vi "NumArray_to_SpdshtStr.vi"(10 "element 2":dbl[](array[numeric]), 11 "element":dbl[](array[numeric])) -> (1 "concatenated string":string, 2 "XY Graph":T1(graph))   [LabVIEW 2015]
panel:
  in  "delimiter (Tab) 2":string
  in  "Column headers":string[](array[string])
  out "spreadsheet string":string
  in  "format string":string
  in  "delimiter (Tab)":string
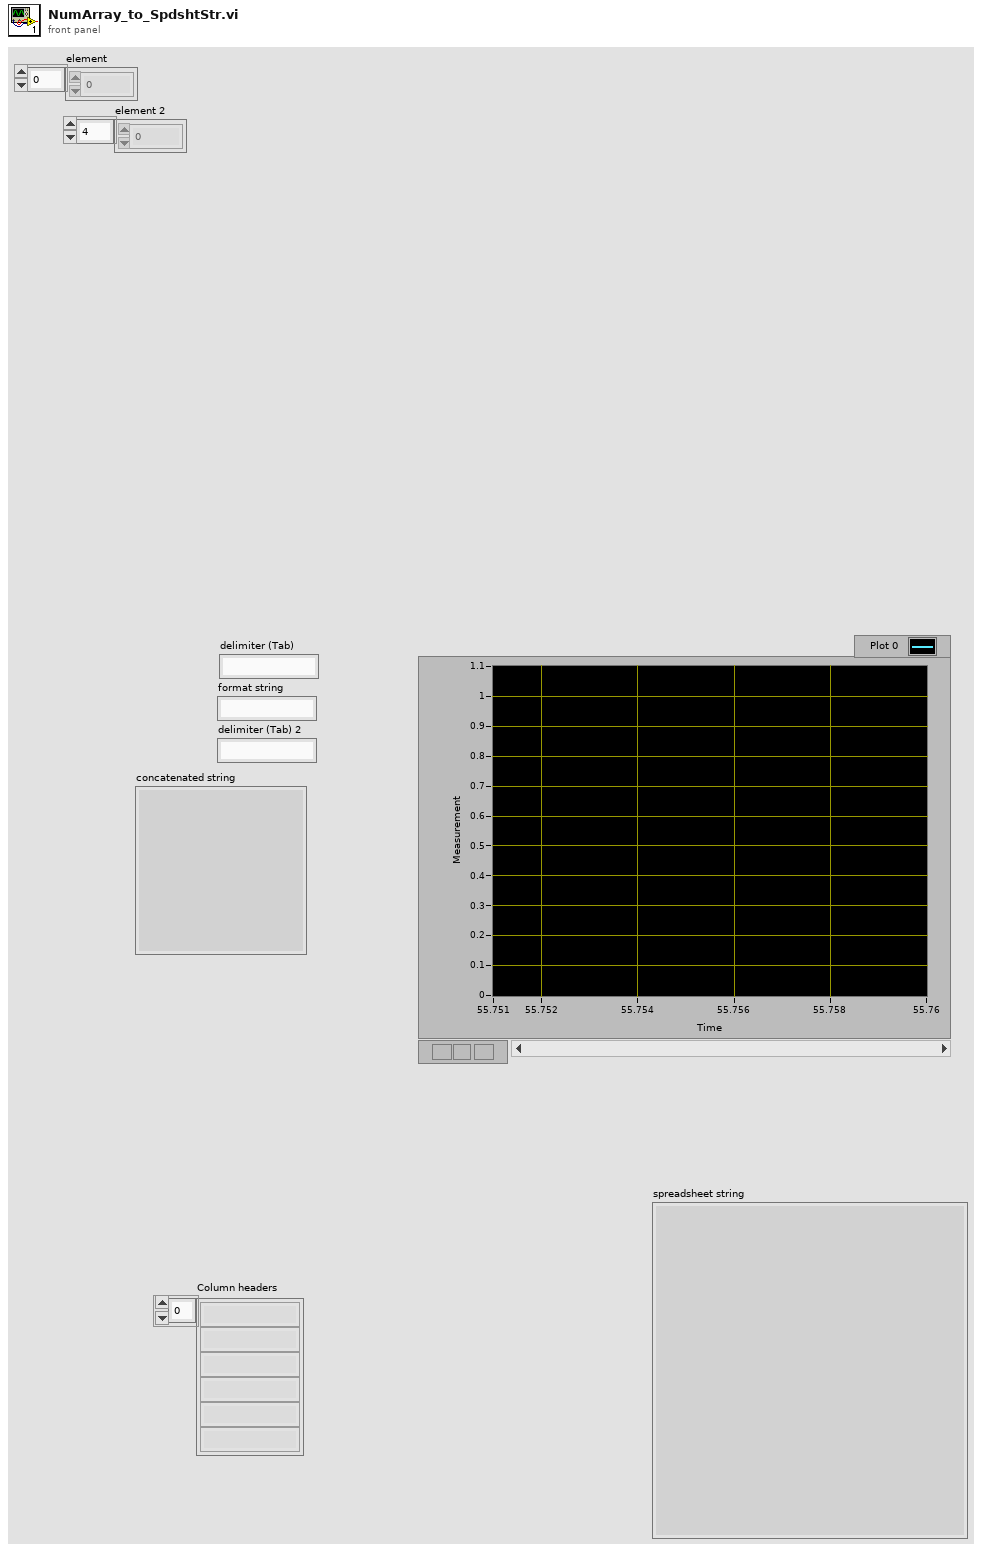
[diagram p1: front panel]
types:
  T1 = cluster{"Measurement Data":dbl[], "Converted Numeric Array":dbl[]}
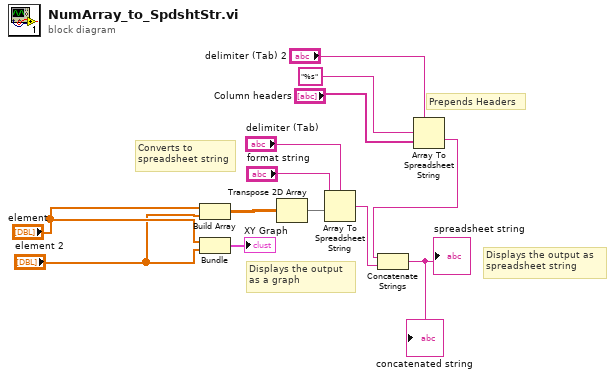
[diagram p0: block diagram]
diagram:
  # "Displays the output as \nspreadsheet string"
  # "Prepends Headers"
  # "Converts to \nspreadsheet string"
  # "Displays the output \nas a graph"
  n1 = Build Array("element", "element 2") -> (w10:dbl[][])
  n2 = Bundle("element"="element", "element 2"="element 2") -> (→"XY Graph":cluster{"element":dbl[], "element 2":dbl[]})  [unwired: 1 in]
  n3 = Transpose 2D Array(2D array=w10) -> (transposed array=w9:dbl[][])
  n4 = Array To Spreadsheet String(delimiter (Tab)="delimiter (Tab)", array=w9, 3:"format string") -> (spreadsheet string=w5:string)
  n5 = Array To Spreadsheet String(delimiter (Tab)="delimiter (Tab) 2", array="Column headers", 3:"%s" ("format string")) -> (spreadsheet string=w6:string)
  n6 = Concatenate Strings(w6, w5) -> (→"spreadsheet string" →"concatenated string":string)
